vi "Export Rejected serials.vi"(8 "error in (no error)":errorcluster, 11 "REF":T1) -> (0 "error out":errorcluster, 2 "Success?":bool, 3 "REF OUT":T1)   [LabVIEW 2024]
uses:
  CTRLS/REF.ctl
  CTRLS/Main Tabs.ctl
  CTRLS/Open Batch Data.ctl
  CTRLS/DM_Data.ctl
  CTRLS/run statistics.ctl
  CTRLS/System settings.ctl
  CTRLS/Printer Message settings.ctl
  CTRLS/Serials DB Operations Enum.ctl
  CTRLS/Serial status Enum.ctl
  <vilib>/Utility/file.llb/Write Delimited Spreadsheet (string).vi
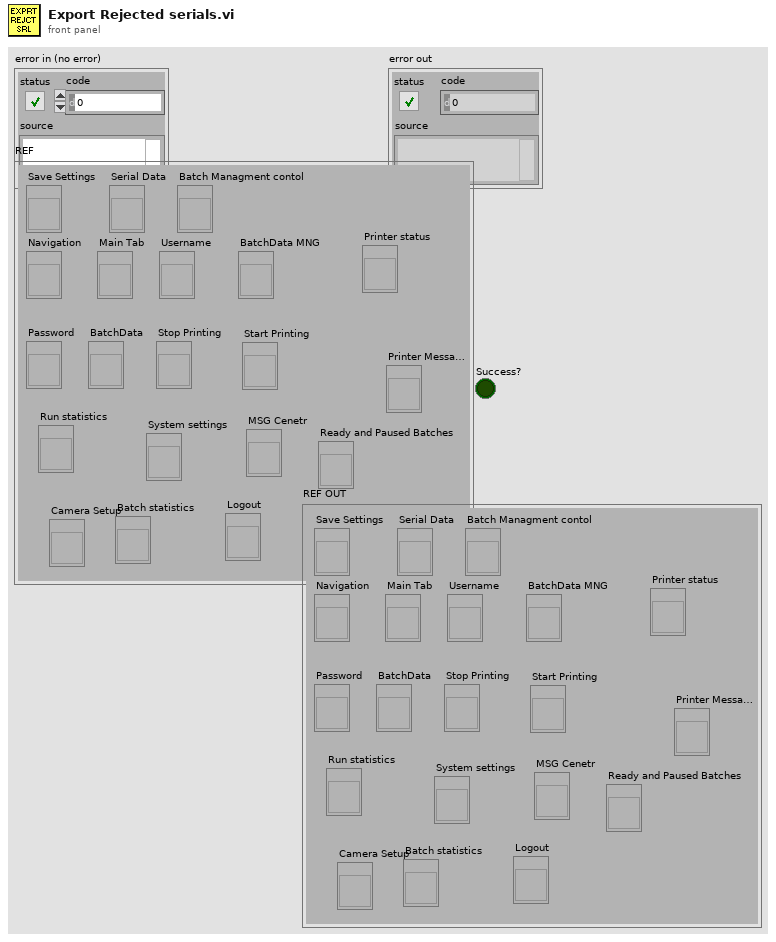
[diagram p1: front panel]
types:
  T1 = typedef "REF.ctl" = cluster{"Save Settings":refnum<vi>, "Navigation":refnum<vi>, "Main Tab":refnum<vi>, "Password":refnum<vi>, "BatchData":refnum<vi>, "Serial Data":refnum<vi>, "Username":refnum<vi>, "Stop Printing":refnum<vi>, "Run statistics":refnum<vi>, "System settings":refnum<vi>, "Batch Managment contol":refnum<vi>, "Start Printing":refnum<vi>, "BatchData MNG":refnum<vi>, "MSG Cenetr":refnum<vi>, "Printer status":refnum<vi>, "Printer Message Config":refnum<vi>, "Ready and Paused Batches":refnum<vi>, "Camera Setup":refnum<vi>, "Batch statistics":refnum<vi>, "Logout":refnum<vi>}
  T2 = typedef "Serial status Enum.ctl" = enum16{"NOT USED", "PRINTED", "ACCEPTED", "REJECTED"}
  T3 = typedef "Serials DB Operations Enum.ctl" = enum16{"Update serial verify status", "Get serials Based on Status", "Insert serials", "Update serial print status", "Get all Batch Serials", "Get Serial Status"}
  T4 = typedef "System settings.ctl" = cluster{"Machine IP":string, "Camera IP":string, "Printer IP":string, "Scanner settings":string, "Server Path":path, "Sending Port":u32, "Recieveing Port":u32}
  T5 = typedef "Open Batch Data.ctl" = cluster{"Batch Name":string, "Batch Number":string, "GTIN":string, "Expiry Date":string, "MFG Date":string}
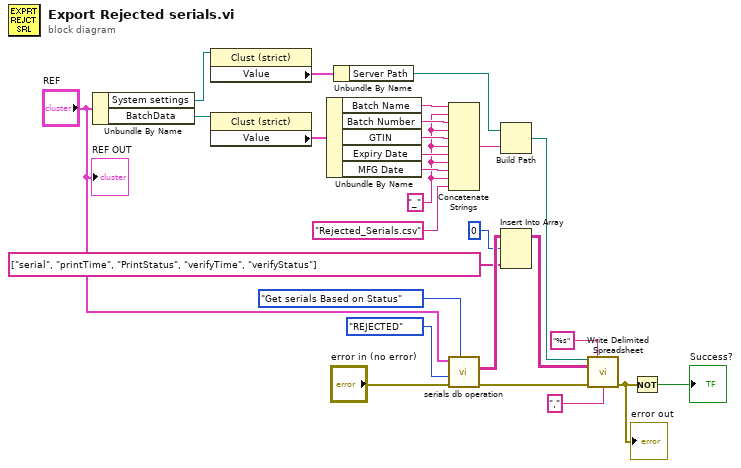
[diagram p0: block diagram]
diagram:
  w11 = "_" ("string")
  n1 = Unbundle By Name("REF") -> ("System settings"=w27:refnum<vi>, "BatchData"=w25:refnum<vi>)
  n2 = property class="Clust (strict)"(reference=w27) -> ("Value"=w26:T4)  [unwired: 1 in, 2 out]
  n3 = property class="Clust (strict)"(reference=w25) -> ("Value"=w17:T5)  [unwired: 1 in, 2 out]
  n4 = Unbundle By Name(w17) -> ("Batch Name"=w16:string, "Batch Number"=w15:string, "GTIN"=w14:string, "Expiry Date"=w13:string, "MFG Date"=w12:string)
  n5 = Unbundle By Name(w26) -> ("Server Path"=w9:path)
  n6 = Concatenate Strings(w16, w11, w15, w11, w14, w11, w13, w11, w12, w11, "Rejected_Serials.csv" ("string")) -> (w8:string)
  n7 = call "serials db operation.vi"("SRL DB OP"=Serials_DB_Operations_Enum."Get serials Based on Status", "error in (no error)"="error in (no error)", "Status"=Serial_status_Enum."REJECTED", "REF"="REF") -> ("error out"=w6:errorcluster, "Fetched Serials"=w21:string[][])  [unwired: 4 in, 2 out]
  n8 = Build Path(base path=w9, name or relative path=w8) -> (appended path=w7:path)
  n9 = Insert Into Array(array=w21, index (row)=0, new element=string[] ["serial", "printTime", "PrintStatus", "verifyTime", "verifyStatus"] ("new element/subarray")) -> (w18:string[][])  [unwired: 1 in]
  n10 = call-poly <vilib>:"Write Delimited Spreadsheet.vi"("file path (dialog if empty)"=w7, "format (%s)"="%s" ("format (%.3f)"), "2D data"=w18, "error in (no error)"=w6, "delimiter (\\t)"="," ("delimiter (\\t)")) -> ("error out"=w3:errorcluster)  [unwired: 9 in, 1 out]
  "error out" <- w3
  n11 = Not(x=w3) -> (.not. x?=→"Success?":bool)
  "REF OUT" <- "REF"
